vi "Periodic Tasks.vi"() -> ()   [LabVIEW 2011]
doc: "This VI runs in parallel to other tasks. It can contain as many user-defined periodic loops as you need. These can carry out PID or other sorts of timed response."
uses:
  <vilib>/Rock Robotics/SystemInterfaces/Utilities/FPGA_UtilitiesLED State.ctl
  <vilib>/Rock Robotics/SystemInterfaces/Utilities/FPGA_UtilitiesLED Source.ctl
  Robot Global Data.vi
  <vilib>/Rock Robotics/WPI/Relay/WPI_RelayValue.ctl
panel:
  out "Rate 3":dbl
  out "error out 4":errorcluster
  out "Direction 3":bool
  out "Distance 3":dbl
  out "Distance 2":dbl
  out "Direction 2":bool
  out "error out 3":errorcluster
  out "Rate 2":dbl
  out "Rate":dbl
  out "error out 2":errorcluster
  out "I2C":bool
  out "Angular Rate":dbl
  out "Angle":dbl
  out "Direction":bool
  out "Distance":dbl
  # "Speed to move to home"
  # "Target Tracking"
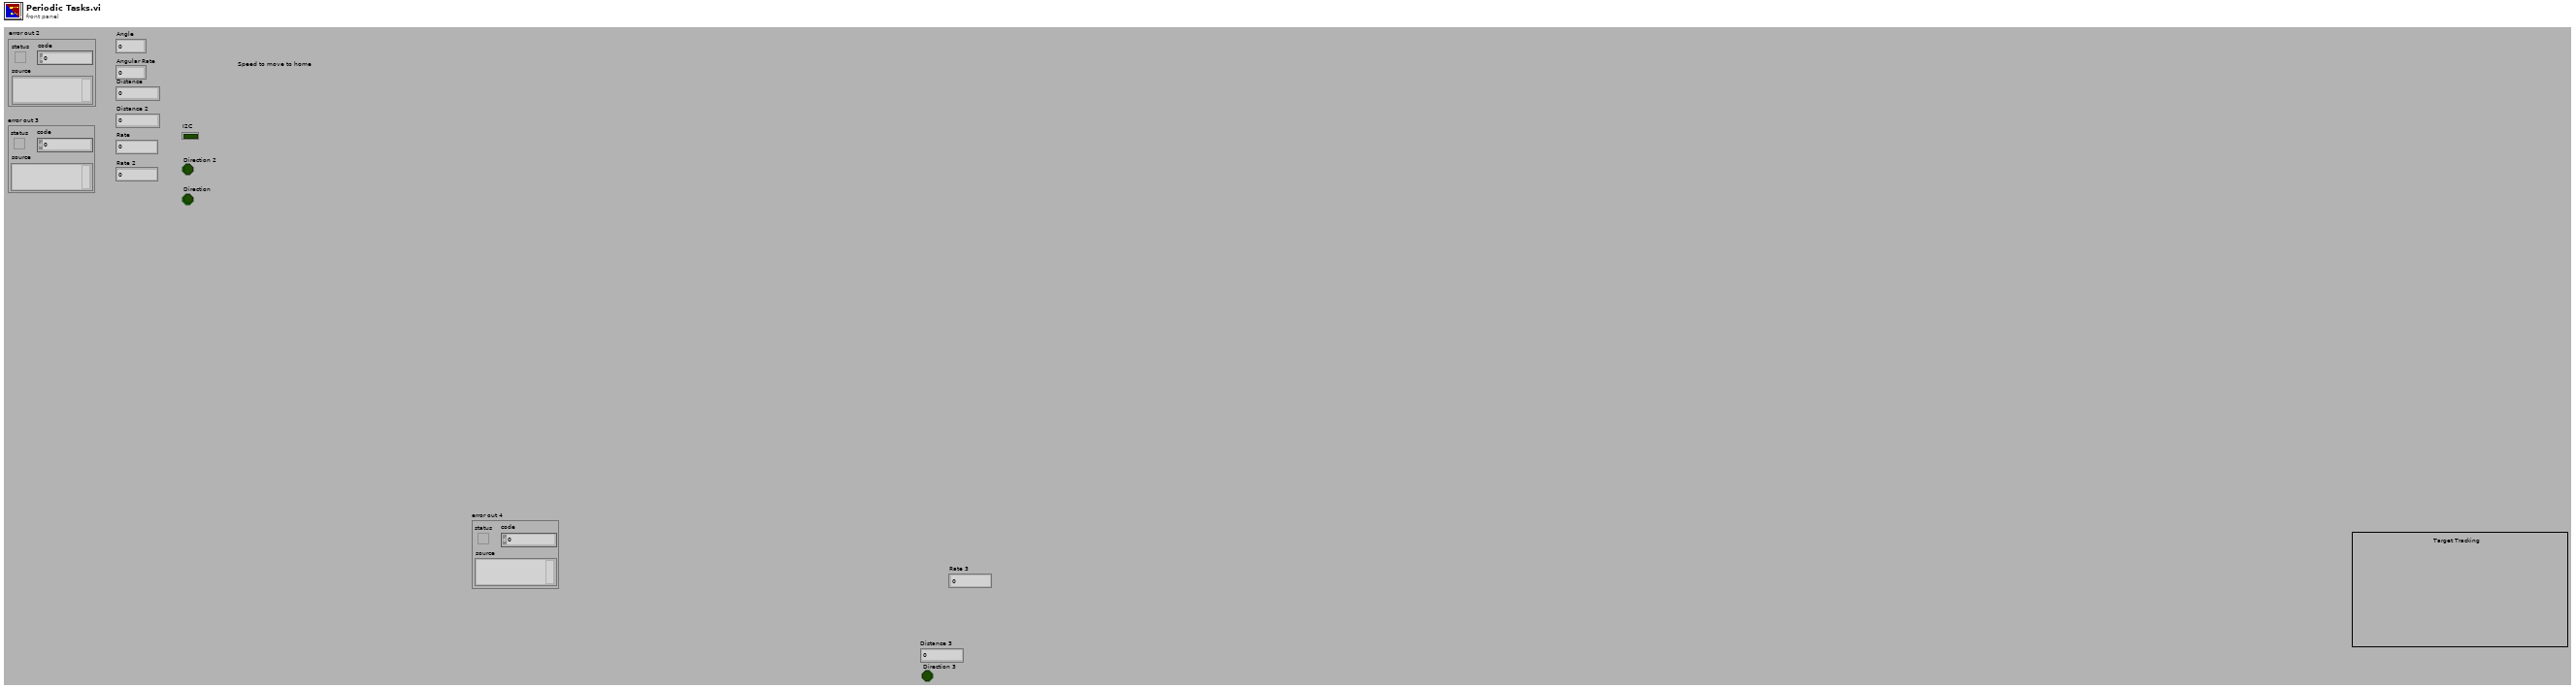
[diagram p1: front panel]
types:
  T1 = typedef "WPI_RelayValue.ctl" = enum16{"Off", "On", "Forward", "Reverse"}
  T2 = typedef "WPI_AnalogChannelDevRef.ctl" = cluster{"DevStatus":errorcluster, "Analog Module":T3, "Analog Channel":T4}
  T3 = typedef "FPGA_TypedefAnalogModule.ctl" = enum16{"Analog Module 1", "Analog Module 2"}
  T4 = typedef "FPGA_AIChannel.ctl" = enum8{"AI 1", "AI 2", "AI 3", "AI 4", "AI 5", "AI 6", "AI 7", "AI 8", "Invalid"}
  T5 = typedef "WPI_EncoderDevRef.ctl" = cluster{"DevStatus":errorcluster, "EncoderIndex":T6, "CounterIndex":T7, "DistancePerCount":dbl, "Decoding Type":T8}
  T6 = typedef "FPGA_EncoderIdx.ctl" = enum8{"Enc 0", "Enc 1", "Enc 2", "Enc 3", "Invalid"}
  T7 = typedef "FPGA_CounterCtrSystemIndex.ctl" = enum8{"Ctr 0", "Ctr 1", "Ctr 2", "Ctr 3", "Ctr 4", "Ctr 5", "Ctr 6", "Ctr 7", "Invalid"}
  T8 = typedef "WPI_EncoderType.ctl" = enum16{"1x", "2x", "4x"}
  T9 = typedef "WPI_RelayDevRef.ctl" = cluster{"DevStatus":errorcluster, "Relay Channel":T10, "Digital Module":T11, "Relay Direction":T12}
  T10 = typedef "FPGA_DIORelayChannel.ctl" = enum8{"Relay 1", "Relay 2", "Relay 3", "Relay 4", "Relay 5", "Relay 6", "Relay 7", "Relay 8", "Invalid"}
  T11 = typedef "FPGA_TypedefDigitalModule.ctl" = enum16{"Digital Module 1", "Digital Module 2"}
  T12 = typedef "WPI_RelayDirection.ctl" = enum16{"Both directions", "Forward only", "Reverse only"}
  T13 = typedef "WPI_GyroDevRef.ctl" = cluster{"DevStatus":errorcluster, "Analog Module":T3, "Analog Channel":T4, "Offset":dbl, "Gain (VoltsPerDegree/Second)":dbl}
  T14 = cluster{"Driver Station Digital Output (1-8)[0]":bool, "Driver Station Digital Output (1-8)[1]":bool, "Driver Station Digital Output (1-8)[2]":bool, "Driver Station Digital Output (1-8)[3]":bool, "Driver Station Digital Output (1-8)[4]":bool, "Driver Station Digital Output (1-8)[5]":bool, "Driver Station Digital Output (1-8)[6]":bool, "Driver Station Digital Output (1-8)[7]":bool, "Driver Station Digital Output (1-8)[8]":bool}
  T15 = typedef "FPGA_UtilitiesLED State.ctl" = enum16{"Off", "On", "Toggle"}
  T16 = typedef "FPGA_UtilitiesLED Source.ctl" = enum16{"User LED", "FPGA LED"}
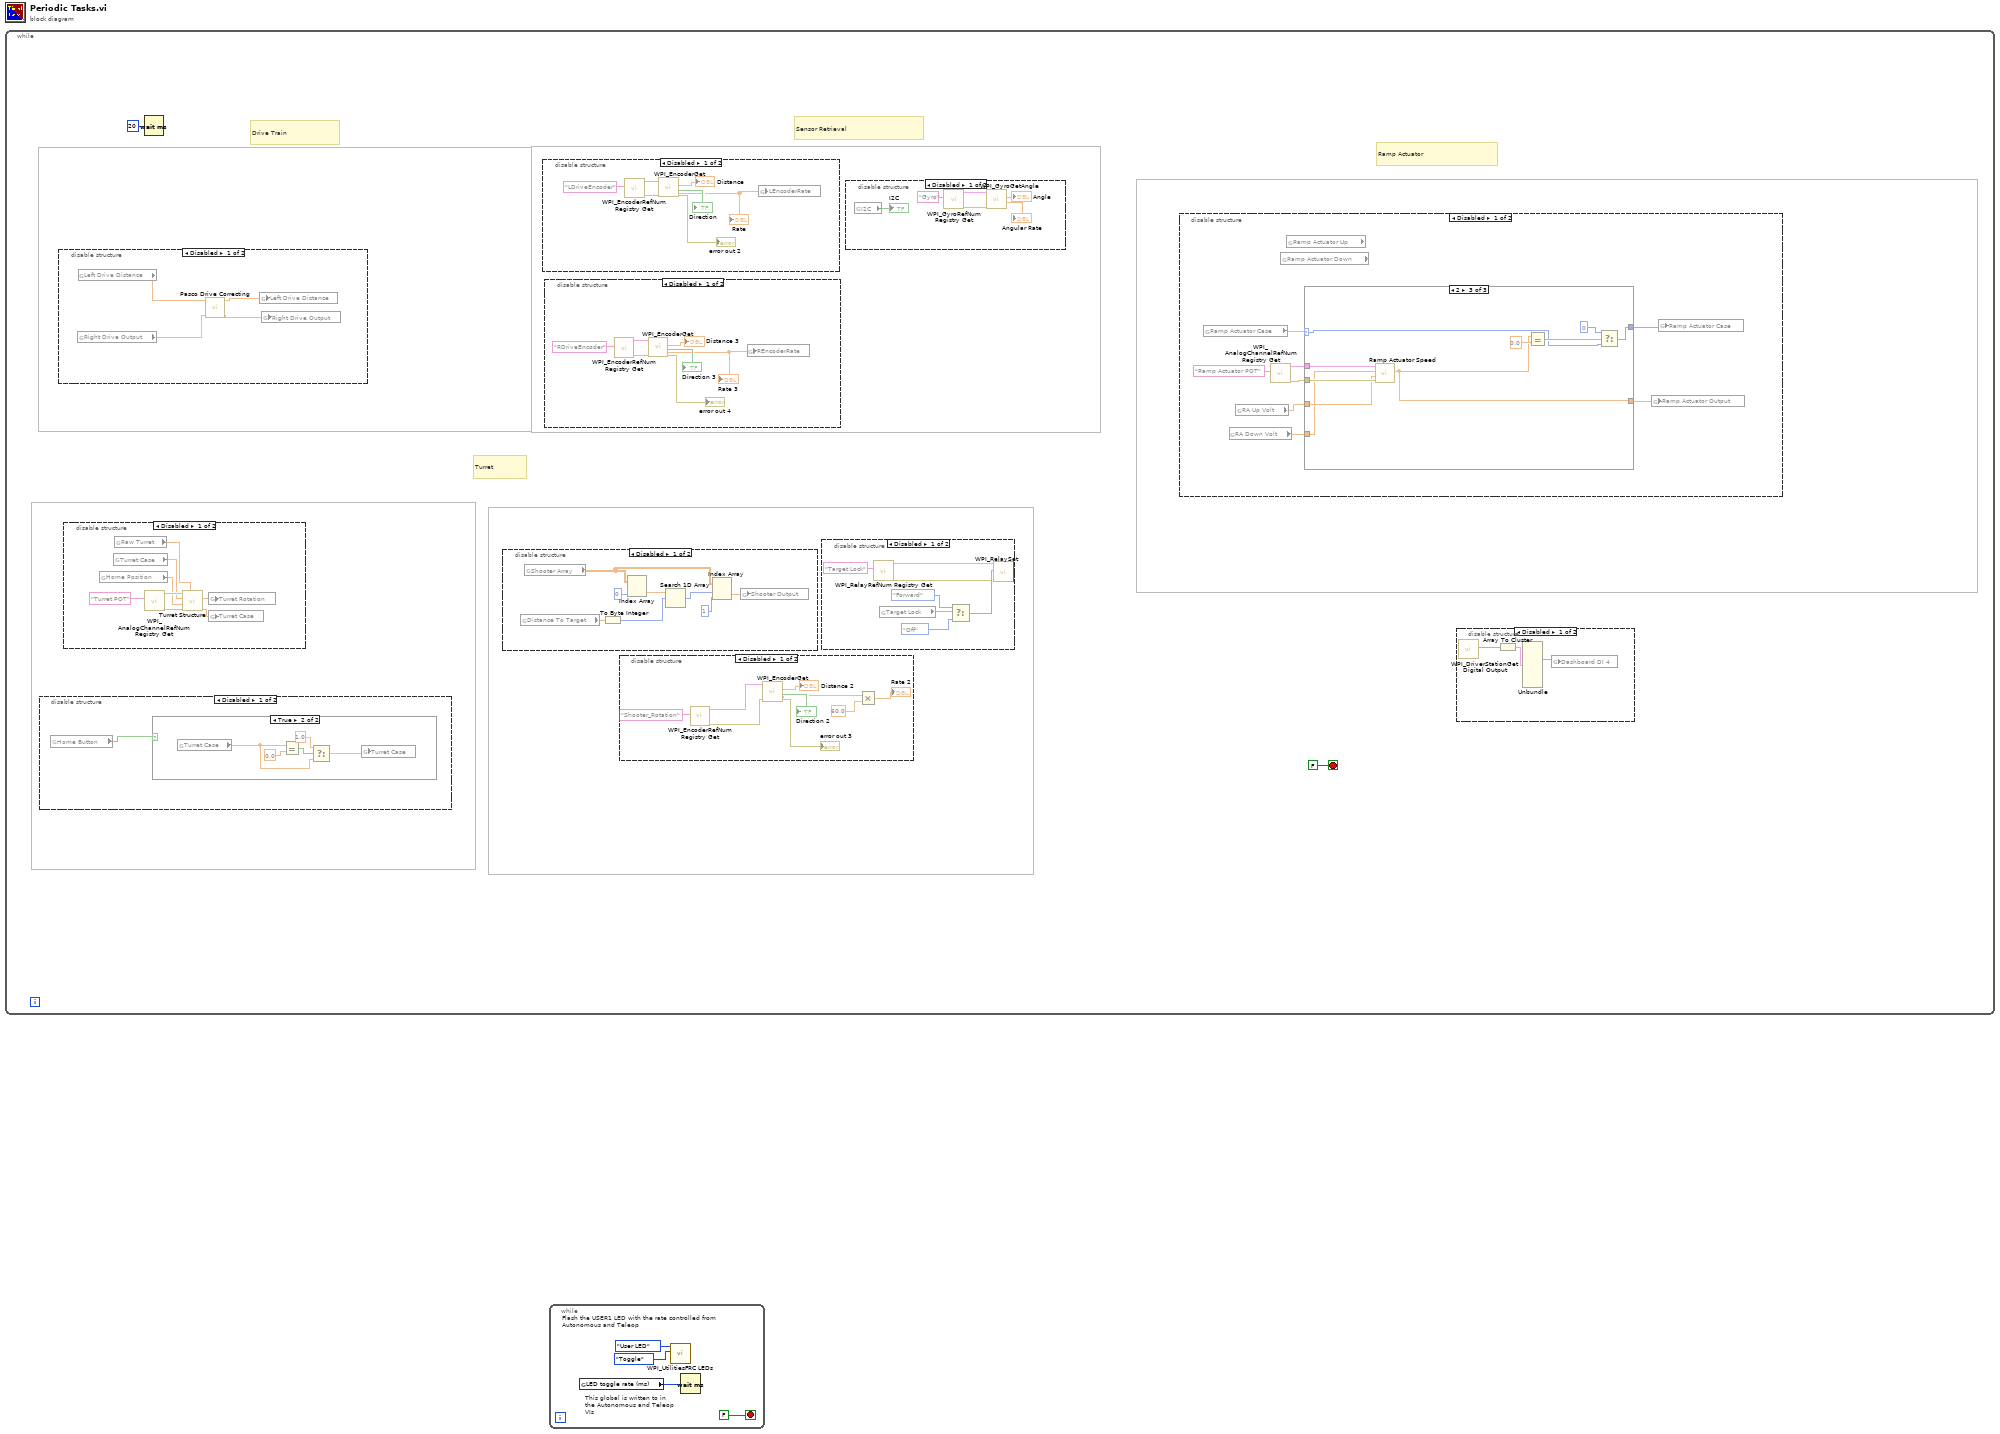
[diagram p0: block diagram]
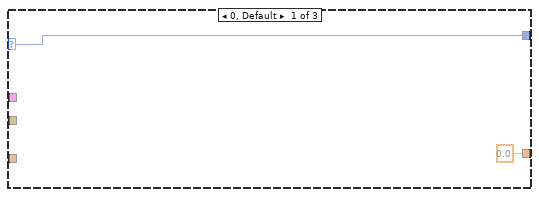
[diagram p3: hidden frame]
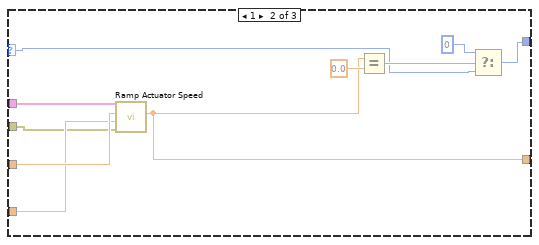
[diagram p4: hidden frame]
diagram:
  n1 = while {
    stop <- FALSE stop-if-true
    # "Sensor Retrieval"
    # "Turret"
    # "Drive Train"
    # "Ramp Actuator"
    n2 = disable-structure shown="Disabled" {
      frame Disabled {
        n3 = global read "Robot Global Data.vi" "Home Button"() -> (w40:bool)
        n4 = case shown="True" w40 {
          frame False {
          }
          frame True {
            n5 = global read "Robot Global Data.vi" "Turret Case"() -> (w42:dbl)
            n6 = Equal?(x=w42, y=0.0) -> (x = y?=w44:bool)
            n7 = Select(t=1.0, s=w44, f=w42) -> (s? t:f=w41:dbl)
            n8 = global write "Robot Global Data.vi" "Turret Case"(w41) -> ()
          }
        }
      }
      frame Enabled {
      }
    }
    n9 = disable-structure shown="Disabled" {
      frame Disabled {
        n10 = global read "Robot Global Data.vi" "Right Drive Output"() -> (w64:dbl)
        n11 = global read "Robot Global Data.vi" "Left Drive Distance"() -> (w65:dbl)
        n12 = call "Pasco Drive Correcting.vi"("RightDriveOutput"=w64, "LeftDriveOutput"=w65) -> ("RightDriveOutput"=w62:dbl, "LeftDriveOutput"=w63:dbl)  [unwired: 8 in]
        n13 = global write "Robot Global Data.vi" "Left Drive Distance"(w63) -> ()
        n14 = global write "Robot Global Data.vi" "Right Drive Output"(w62) -> ()
      }
      frame Enabled {
      }
    }
    n15 = disable-structure shown="Disabled" {
      frame Disabled {
        n16 = global read "Robot Global Data.vi" "Home Position"() -> (w49:dbl)
        n17 = global read "Robot Global Data.vi" "Turret Case"() -> (w50:dbl)
        n18 = global read "Robot Global Data.vi" "Raw Turret"() -> (w48:dbl)
        n19 = call <vilib>:"WPI_AnalogChannelRefNum Registry Get.vi"("refnum name"="Turret POT") -> ("error out"=w51:errorcluster, "AIDeviceRef"=w52:T2)  [unwired: 9 in]
        n20 = call "Turret Structure.vi"("Raw Turret"=w48, "error in (no error)"=w51, "Home postion"=w49, "Turret Case"=w50, "AIDeviceRef"=w52) -> ("Turret Case Output"=w46:dbl, "Turret Output"=w47:dbl)  [unwired: 5 in]
        n21 = global write "Robot Global Data.vi" "Turret Rotation"(w47) -> ()
        n22 = global write "Robot Global Data.vi" "Turret Case"(w46) -> ()
      }
      frame Enabled {
      }
    }
    n23 = Wait (ms)(milliseconds to wait=u32 20) -> ()  [unwired: 1 out]
    n24 = disable-structure shown="Disabled" {
      frame Disabled {
        n25 = global read "Robot Global Data.vi" "Distance To Target"() -> (w59:dbl)
        n26 = global read "Robot Global Data.vi" "Shooter Array"() -> (w57:dbl[][])
        n27 = To Byte Integer(number=w59) -> (8bit integer=w58:i8)
        n28 = Index Array(array=w57, index (col)=0 ("disabled index (col)")) -> (element=w60:dbl[])  [unwired: 1 in]
        n29 = Search 1D Array(1D array=w60, element=w58) -> (index of element=w56:i32)  [unwired: 1 in]
        n30 = Index Array(array=w57, index (row)=w56, index (col)=1 ("disabled index (col)")) -> (element=w54:dbl)
        n31 = global write "Robot Global Data.vi" "Shooter Output"(w54) -> ()
      }
      frame Enabled {
      }
    }
    n32 = disable-structure shown="Disabled" {
      frame Disabled {
        n33 = call <vilib>:"WPI_EncoderRefNum Registry Get.vi"("refnum name"="LDriveEncoder") -> ("error out"=w80:errorcluster, "EncoderDevRef"=w79:T5)  [unwired: 9 in]
        n34 = call <vilib>:"WPI_EncoderGet.vi"("error in (no error)"=w80, "EncoderDevRef"=w79) -> ("error out"=→"error out 2":errorcluster, "Direction"=→"Direction":bool, "Distance"=→"Distance":dbl, "Rate"=w76:dbl)  [unwired: 4 in, 2 out]
        "Rate" <- w76
        n35 = global write "Robot Global Data.vi" "LEncoderRate"(w76) -> ()
      }
      frame Enabled {
      }
    }
    n36 = disable-structure shown="Disabled" {
      frame Disabled {
        n37 = call <vilib>:"WPI_EncoderRefNum Registry Get.vi"("refnum name"="RDriveEncoder") -> ("error out"=w73:errorcluster, "EncoderDevRef"=w72:T5)  [unwired: 9 in]
        n38 = call <vilib>:"WPI_EncoderGet.vi"("error in (no error)"=w73, "EncoderDevRef"=w72) -> ("error out"=→"error out 4":errorcluster, "Direction"=→"Direction 3":bool, "Distance"=→"Distance 3":dbl, "Rate"=w69:dbl)  [unwired: 4 in, 2 out]
        "Rate 3" <- w69
        n39 = global write "Robot Global Data.vi" "REncoderRate"(w69) -> ()
      }
      frame Enabled {
      }
    }
    n40 = disable-structure shown="Disabled" {
      frame Disabled {
        n41 = call <vilib>:"WPI_EncoderRefNum Registry Get.vi"("refnum name"="Shooter_Rotation") -> ("error out"=w89:errorcluster, "EncoderDevRef"=w90:T5)  [unwired: 9 in]
        n42 = call <vilib>:"WPI_EncoderGet.vi"("error in (no error)"=w89, "EncoderDevRef"=w90) -> ("error out"=→"error out 3":errorcluster, "Direction"=→"Direction 2":bool, "Distance"=→"Distance 2":dbl, "Rate"=w93:dbl)  [unwired: 4 in, 2 out]
        n43 = Multiply(x=w93, y=60.0) -> (x*y=→"Rate 2":dbl)
      }
      frame Enabled {
      }
    }
    n44 = disable-structure shown="Disabled" {
      frame Disabled {
        n45 = call <vilib>:"WPI_RelayRefNum Registry Get.vi"("refnum name"="Target Lock") -> ("error out"=w3:errorcluster, "RelayDevRef"=w4:T9)  [unwired: 9 in]
        n46 = global read "Robot Global Data.vi" "Target Lock"() -> (w9:bool)
        n47 = Select(t=WPI_RelayValue."Forward" ("RelayValue"), s=w9, f=WPI_RelayValue."Off" ("RelayValue")) -> (s? t:f=w6:T1)
        n48 = call <vilib>:"WPI_RelaySet.vi"("error in (no error)"=w3, "RelayValue"=w6, "RelayDevRef"=w4) -> ()  [unwired: 7 in, 2 out]
      }
      frame Enabled {
      }
    }
    n49 = disable-structure shown="Disabled" {
      frame Disabled {
        n50 = global read "Robot Global Data.vi" "I2C"() -> (→"I2C":bool)
        n51 = call <vilib>:"WPI_GyroRefNum Registry Get.vi"("refnum name"="Gyro") -> ("error out"=w87:errorcluster, "GyroDevRef"=w88:T13)  [unwired: 9 in]
        n52 = call <vilib>:"WPI_GyroGetAngle.vi"("error in (no error)"=w87, "GyroDevRef"=w88) -> ("Angular Rate"=→"Angular Rate":dbl, "Angle"=→"Angle":dbl)  [unwired: 6 in, 2 out]
      }
      frame Enabled {
      }
    }
    n53 = disable-structure shown="Disabled" {
      frame Disabled {
        n54 = global read "Robot Global Data.vi" "Ramp Actuator Case"() -> (w17:dbl)
        n55 = global read "Robot Global Data.vi" "RA Down Volt"() -> (w12:dbl)
        n56 = global read "Robot Global Data.vi" "RA Up Volt"() -> (w13:dbl)
        n57 = call <vilib>:"WPI_AnalogChannelRefNum Registry Get.vi"("refnum name"="Ramp Actuator POT") -> ("error out"=w10:errorcluster, "AIDeviceRef"=w11:T2)  [unwired: 9 in]
        n58 = global read "Robot Global Data.vi" "Ramp Actuator Down"() -> ()  [unwired: 1 out]
        n59 = global read "Robot Global Data.vi" "Ramp Actuator Up"() -> ()  [unwired: 1 out]
        n60 = case shown="2" w17 {
          selector: w17 -> [w19 w23 w34]
          tunnel: [w19 w20 w36] -> w16
          tunnel: [0.0 ("f") w21 w35] -> w14
          tunnel: w13 -> [_ w29 w31]
          tunnel: w12 -> [_ w28 w30]
          tunnel: w11 -> [_ w27 w33]
          tunnel: w10 -> [_ w26 w32]
          frame 0, Default {
          }
          frame 1 {
            n61 = call "Ramp Actuator Speed.vi"("error in (no error)"=w26, "RA Down Volt"=w28, "RA Up Volt"=w29, "AIDeviceRef"=w27) -> ("Ramp Actuator Ouput"=w21:dbl)  [unwired: 7 in]
            n62 = Equal?(x=w21, y=0.0) -> (x = y?=w24:bool)
            n63 = Select(t=0, s=w24, f=w23) -> (s? t:f=w20:i32)
          }
          frame 2 {
            n64 = call "Ramp Actuator Speed.vi"("error in (no error)"=w32, "RA Down Volt"=w31, "RA Up Volt"=w30, "AIDeviceRef"=w33) -> ("Ramp Actuator Ouput"=w35:dbl)  [unwired: 7 in]
            n65 = Equal?(x=w35, y=0.0) -> (x = y?=w38:bool)
            n66 = Select(t=0, s=w38, f=w34) -> (s? t:f=w36:i32)
          }
        }
        n67 = global write "Robot Global Data.vi" "Ramp Actuator Output"(w14) -> ()
        n68 = global write "Robot Global Data.vi" "Ramp Actuator Case"(w16) -> ()
      }
      frame Enabled {
      }
    }
    n69 = disable-structure shown="Disabled" {
      frame Disabled {
        n70 = call <vilib>:"WPI_DriverStationGet Digital Output.vi"() -> ("Driver Station Digital Output (1-8)"=w68:bool[])  [unwired: 10 in, 1 out]
        n71 = Array To Cluster(array=w68) -> (cluster=w67:T14)
        n72 = Unbundle(w67) -> ("Driver Station Digital Output (1-8)[3]"=w66:bool)  [unwired: 8 out]
        n73 = global write "Robot Global Data.vi" "Dashboard DI 4"(w66) -> ()
      }
      frame Enabled {
      }
    }
  }
  n74 = while {
    stop <- FALSE stop-if-true
    # "This global is written to in the Autonomous and Teleop VIs"
    # "Flash the USER1 LED with the rate controlled from Autonomous and Teleop"
    n75 = global read "Robot Global Data.vi" "LED toggle rate (ms)"() -> (w98:u32)
    n76 = call <vilib>:"WPI_UtilitiesFRC LEDs.vi"("State"=FPGA_UtilitiesLED_State."Toggle", "LED Type"=FPGA_UtilitiesLED_Source."User LED") -> ()  [unwired: 1 in, 9 out]
    n77 = Wait (ms)(milliseconds to wait=w98) -> ()  [unwired: 1 out]
  }
